vi "Engine-Out.vi"(8 "error in (no error)":errorcluster, 11 "DSI Reference":refnum<class "DCM-DSI.lvclass">) -> (0 "error out":errorcluster, 3 "DSI Reference":refnum<class "DCM-DSI.lvclass">)   [LabVIEW 2016, in "DSI-RT.lvlib"]
uses:
  DSI-RT.lvlib
  Classes/DCM-DSI/DCM-DSI.lvclass
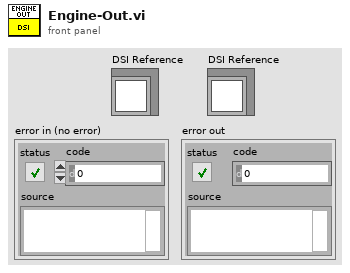
[diagram p1: front panel]
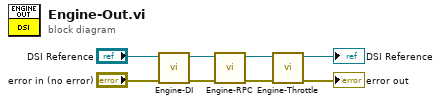
[diagram p0: block diagram]
diagram:
  n1 = call "Engine-DI.vi"("Error In"="error in (no error)", "DSI Reference"="DSI Reference") -> ("Error Out"=w5:errorcluster, "DSI Reference"=w6:refnum<class "DCM-DSI.lvclass">)  [unwired: 8 in]
  n2 = call "Engine-RPC.vi"("Error In"=w5, "DSI Reference"=w6) -> ("Error Out"=w3:errorcluster, "DSI Reference"=w4:refnum<class "DCM-DSI.lvclass">)  [unwired: 8 in]
  n3 = call "Engine-Throttle.vi"("Error In"=w3, "DSI Reference"=w4) -> ("Error Out"=→"error out":errorcluster, "DSI Reference"=→"DSI Reference":refnum<class "DCM-DSI.lvclass">)  [unwired: 8 in]
